vi "DataEvent-Treatment.vi"(8 "error in (no error)":errorcluster, 9 "data":variant, 10 "command":string, 11 "Control-Server in":refnum<class "Control-Server.lvclass">) -> (0 "error out":errorcluster, 3 "Control-Server out":refnum<class "Control-Server.lvclass">)   [LabVIEW 2020, in "Control-Server.lvclass"]
uses:
  Control-Server.lvclass
  dependecies/ControlsVIs/Clusters-def/SERVER-Commands.ctl
  Delay Line/DelayLine.lvclass
  dependecies/ControlsVIs/Clusters-def/DL-Reply-to-Connect.ctl
  dependecies/ControlsVIs/Clusters-def/Message types.ctl
  dependecies/ControlsVIs/Clusters-def/Standard Command.ctl
  Message/Message.lvclass
  dependecies/globalVarII.vi
  GeneralFunctionality/GeneralFunctionality.lvclass
  C:/dev/TRANCON/Classes/GeneralFunctionality/GeneralFunctionality.lvclass
  C:/dev/TRANCON/Classes/Control/Control-Server/Control-Server.lvclass
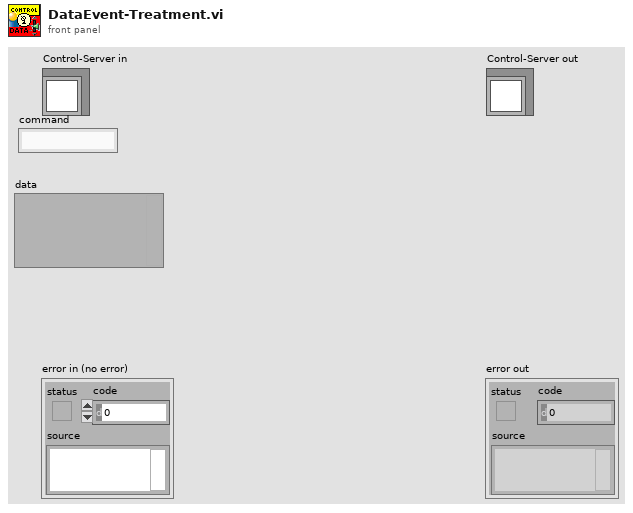
[diagram p1: front panel]
types:
  T1 = typedef "Standard Command.ctl" = cluster{"command":string, "data":variant}
  T2 = typedef "Control-Server.lvclass/SERVER-Commands.ctl" = string
  T3 = typedef "Message types.ctl" = string
  T4 = typedef "DelayLine.lvclass/DL-Reply-to-Connect.ctl" = cluster{"On/Off":bool, "error":errorcluster, "DelayLine.lvclass":refnum<class "DelayLine.lvclass">}
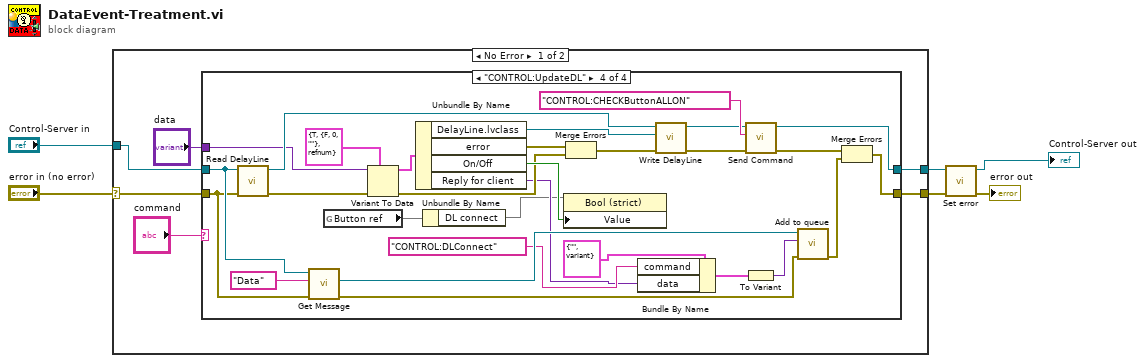
[diagram p0: block diagram]
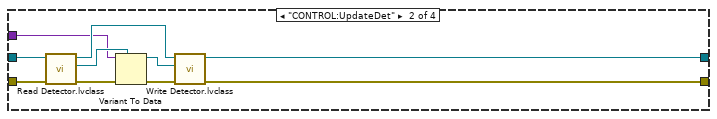
[diagram p3: hidden frame]
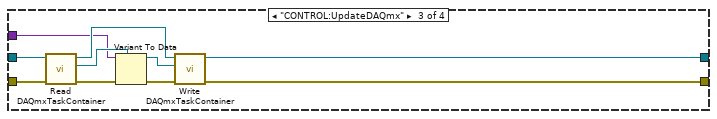
[diagram p4: hidden frame]
diagram:
  n1 = case shown="No Error" "error in (no error)" {
    selector: "error in (no error)" -> [w7 w65]
    tunnel: "Control-Server in" -> [w10 w64]
    tunnel: [w9 w64] -> w4
    tunnel: [w8 w65] -> w2
    frame No Error {
      n2 = case shown="\"CONTROL:UpdateDL\"" "command" {
        tunnel: w10 -> [w14 w21 w31 w42]
        tunnel: w7 -> [w13 w20 w30 w41]
        tunnel: [w14 w18 w28 w60] -> w9
        tunnel: [w13 w17 w27 w38] -> w8
        tunnel: "data" -> [_ w15 w25 w61]
        frame "False", Default {
        }
        frame "CONTROL:UpdateDet" {
          n3 = call "Read Detector.lvclass.vi"("error in (no error)"=w20, "Control in"=w21) -> ("error out"=w22:errorcluster, "Detector.lvclass"=w24:refnum<class "Detector.lvclass">, "Control out"=w19:refnum<class "Control-Server.lvclass">)  [unwired: 7 in]
          n4 = Variant To Data(error in=w22, type=w24, Variant=w15) -> (data=w23:refnum<class "Detector.lvclass">, error out=w16:errorcluster)
          n5 = call "Write Detector.lvclass.vi"("error in (no error)"=w16, "Detector.lvclass"=w23, "Control in"=w19) -> ("error out"=w17:errorcluster, "Control out"=w18:refnum<class "Control-Server.lvclass">)  [unwired: 7 in]
        }
        frame "CONTROL:UpdateDAQmx" {
          n6 = call-dynamic "Read DAQmxTaskContainer.vi"("error in (no error)"=w30, "Control in"=w31) -> ("error out"=w32:errorcluster, "DAQmxTaksContainer_General.lvclass"=w34:refnum<class "DAQmxTaksContainer_General.lvclass">, "Control out"=w29:refnum<class "Control-Server.lvclass">)  [unwired: 7 in]
          n7 = Variant To Data(error in=w32, type=w34, Variant=w25) -> (data=w33:refnum<class "DAQmxTaksContainer_General.lvclass">, error out=w26:errorcluster)
          n8 = call-dynamic "Write DAQmxTaskContainer.vi"("error in (no error)"=w26, "DAQmxTaksContainer_General.lvclass"=w33, "Control in"=w29) -> ("error out"=w27:errorcluster, "Control out"=w28:refnum<class "Control-Server.lvclass">)  [unwired: 7 in]
        }
        frame "CONTROL:UpdateDL" {
          n9 = call "Read DelayLine.vi"("error in (no error)"=w41, "Control in"=w42) -> ("error out"=w62:errorcluster, "Control out"=w63:refnum<class "Control-Server.lvclass">)  [unwired: 7 in, 1 out]
          n10 = call "Get Message.vi"("error in (no error)"=w41, "Message type"=T3 "Data", "GeneralFunctionality en entrée"=w42) -> ("error out"=w40:errorcluster, "Message.lvclass"=w50:refnum<class "Message.lvclass">)  [unwired: 6 in, 1 out]
          n11 = global read "globalVarII.vi" "Button ref"() -> (w36)
          n12 = Variant To Data(error in=w62, type=T4 {"On/Off"=TRUE, "error"={"status"=FALSE, "code"=0, "source"=""}, "DelayLine.lvclass"=refnum}, Variant=w61) -> (data=w56:T4, error out=w52:errorcluster)
          n13 = Unbundle By Name(w56) -> ("DelayLine.lvclass"=w55:refnum<class "DelayLine.lvclass">, "error"=w53:errorcluster, "On/Off"=w54:bool, "Reply for client"=w44:variant)
          n14 = Unbundle By Name(w36) -> ("DL connect"=w35)
          n15 = property class="Bool (strict)"(reference=w35, "Value"=w54) -> ()  [unwired: 1 in, 2 out]
          n16 = Merge Errors(w53, w52) -> (w51:errorcluster)
          n17 = Bundle By Name(cluster=T1 {"command"="", "data"=variant} ("input cluster"), "command"=T2 "CONTROL:DLConnect" ("Commands"), "data"=w44) -> (w48:T1)
          n18 = call "Write DelayLine.vi"("error in (no error)"=w51, "DelayLine.lvclass"=w55, "Control in"=w63) -> ("error out"=w58:errorcluster, "Control out"=w43:refnum<class "Control-Server.lvclass">)  [unwired: 7 in]
          n19 = call "Send Command.vi"("error in (no error)"=w58, "Commands"=T2 "CONTROL:CHECKButtonALLON", "Control en entrée"=w43) -> ("error out"=w39:errorcluster, "Control en sortie"=w60:refnum<class "Control-Server.lvclass">)  [unwired: 7 in]
          n20 = To Variant(anything=w48) -> (Variant=w49:variant)
          n21 = call "Add to queue.vi"("error in (no error)"=w40, "Data"=w49, "Message in"=w50) -> ("error out"=w37:errorcluster)  [unwired: 7 in, 1 out]
          n22 = Merge Errors(w39, w37) -> (w38:errorcluster)
        }
      }
    }
    frame Error {
    }
  }
  n23 = call "Set error.vi"("error in (no error)"=w2, "Control-Server in"=w4) -> ("error out"=→"error out":errorcluster, "Control-Server out"=→"Control-Server out":refnum<class "Control-Server.lvclass">)  [unwired: 8 in]
